vi "PFI-28000-Chan-28144-I_Get Gage.vi"(8 "error in (no error)":errorcluster, 11 "PFI-28000-Chan-28144-I in":refnum<class "PFI-28000-Chan-28144-I.lvclass">) -> (0 "error out":errorcluster, 2 "Gage":T1, 3 "PFI-28000-Chan-28144-I out":refnum<class "PFI-28000-Chan-28144-I.lvclass">)   [LabVIEW 2017, in "PFI-28000-Chan-28144-I.lvclass"]
uses:
  PFI-28000-Chan-28144-I.lvclass
  C:/wc/07143 Precision Filters 28000 Support/Driver/source/Channel/PFI-28000-Channel.lvclass
  PFI-28000-Chan-28144-Gage.ctl
  Utilities/PFI-28000-Utils.lvlib
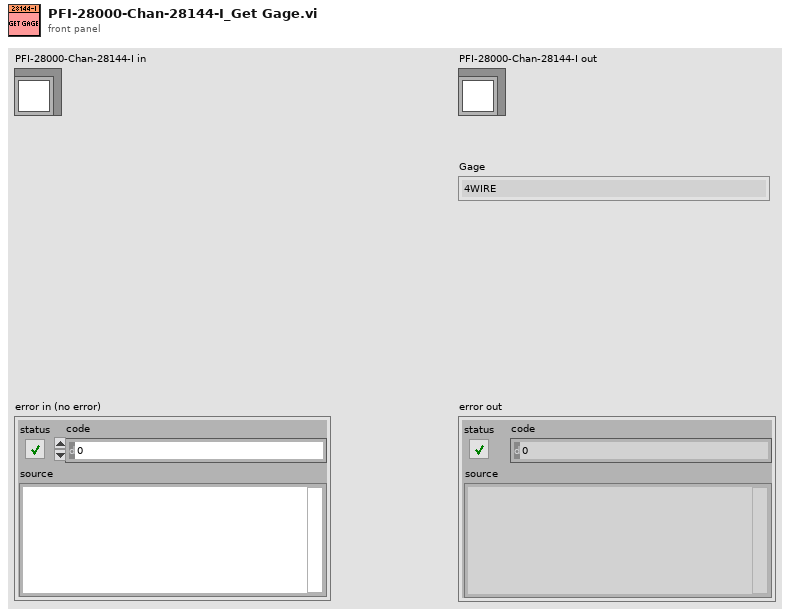
[diagram p1: front panel]
types:
  T1 = typedef "PFI-28000-Chan-28144-I.lvclass/PFI-28000-Chan-28144-Gage.ctl" = enum8{"4WIRE", "2WIRE"}
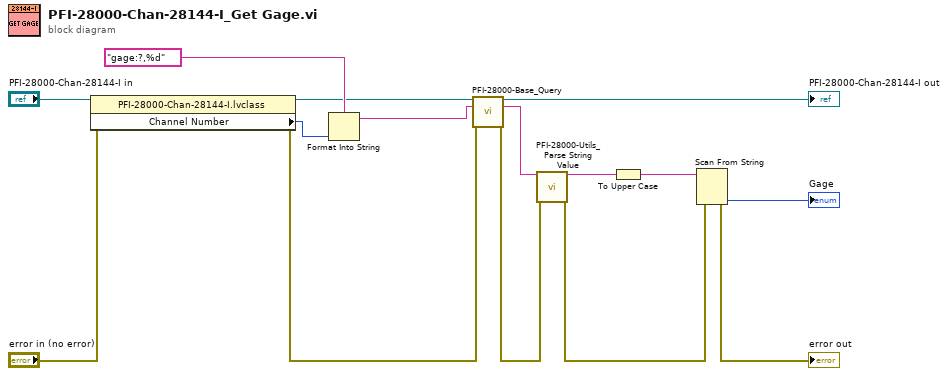
[diagram p0: block diagram]
diagram:
  n1 = property class="PFI-28000-Chan-28144-I.lvclass"(reference="PFI-28000-Chan-28144-I in", error in="error in (no error)") -> (reference out=w8:refnum<class "PFI-28000-Chan-28144-I.lvclass">, error out=w7:errorcluster, "Channel Number"=w13:i32)
  n2 = Format Into String(format string="gage:?,%d" ("empty string"), w13) -> (resulting string=w9:string)  [unwired: 2 in, 1 out]
  n3 = call-dynamic "PFI-28000-Base_Query.vi"("PFI-28000-Base in"=w8, "Command"=w9, "error in (no error)"=w7) -> ("PFI-28000-Base out"=→"PFI-28000-Chan-28144-I out":refnum<class "PFI-28000-Chan-28144-I.lvclass">, "Response"=w3:string, "error out"=w5:errorcluster)  [unwired: 9 in, 1 out]
  n4 = call "PFI-28000-Utils_Parse String Value.vi"("String"=w3, "error in (no error)"=w5) -> ("String Value"=w2:string, "error out"=w4:errorcluster)  [unwired: 11 in, 1 out]
  n5 = To Upper Case(1:w2) -> (0:w1:string)
  n6 = Scan From String(input string=w1, error in=w4) -> (error out=→"error out":errorcluster, output 1=→"Gage":T1)  [unwired: 3 in, 2 out]
